vi "Fpga-Top-Level.vi"() -> ()   [LabVIEW 2016]
uses:
  <vilib>/Platform/TimedLoop/XDataNode/timing_clust.ctl
  <vilib>/Platform/TimedLoop/XDataNode/nitl_modes.ctl
  <vilib>/Platform/TimedLoop/XDataNode/wakeup.ctl
  <vilib>/rvi/Emulation/niFpgaSctlEmulationGetInTimedLoop.vi
  <vilib>/rvi/Emulation/niFpgaEmulationReportErrorSimple.vi
  <vilib>/rvi/Emulation/niFpgaGetClockAttributes.vi
  <vilib>/rvi/Emulation/niFpgaCriticalErrorInLSC.vi
  <vilib>/rvi/interface/RandomDataEmulation/niFpgaRandomDataHandleErrors.vi
  <vilib>/Platform/TimedLoop/XDataNode/XDataNode.xnode
  <vilib>/rvi/DataTransferAndStorage/Container/XNode/niFpgaContainer.xnode
  <vilib>/rvi/interface/RandomDataEmulation/nirviRandomDataFpgaReadWriteTemplate.vi
  <vilib>/Platform/TimedLoop/XDataNode/XDNodeRunTimeDep.lvlib
panel:
  out "Seconds":u32 format="%.0x"
  out "MsgType":u8
  out "MsgLen (16)":u16
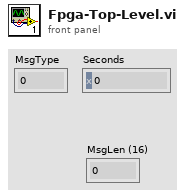
[diagram p1: front panel]
types:
  T1 = typedef "XDNodeRunTimeDep.lvlib/timing_clust.ctl" = cluster{"Expected End [f-1]":u64, "Actual End [f-1]":u64, "Finished Late? [f-1]":bool, "Expected End [i-1]":u64, "Actual End [i-1]":u64, "Finished Late? [i-1]":bool, "Expected Start [i]":u64, "Actual Start [i]":u64, "Expected Start [f]":u64, "Actual Start [f]":u64, "Source Name":string, "Structure Name":string, "Period":i64, "Deadline":i64, "Offset":i64, "Start":i64, "Priority":i32, "Timeout":i32, "Mode":T2, "Wakeup Reason":T3, "Error":errorcluster, "Source Type":string, "Secondary Source Type":string, "Global End Time":u64, "Global Start Time":u64, "Frame Duration":u64, "Iteration Duration":u64, "Assigned CPU":i32, "I/O Scan Engine Mode":u32}
  T2 = typedef "XDNodeRunTimeDep.lvlib/nitl_modes.ctl" = enum32{"No Change", "Process missed periods, maintain original phase", "Discard missed periods, maintain original phase", "Process missed periods, ignore original phase", "Discard missed periods, ignore original phase"}
  T3 = typedef "XDNodeRunTimeDep.lvlib/wakeup.ctl" = enum32{"Normal", "Aborted", "Asynchronous wakeup", "Timing source error", "Timed loop error", "Timeout"}
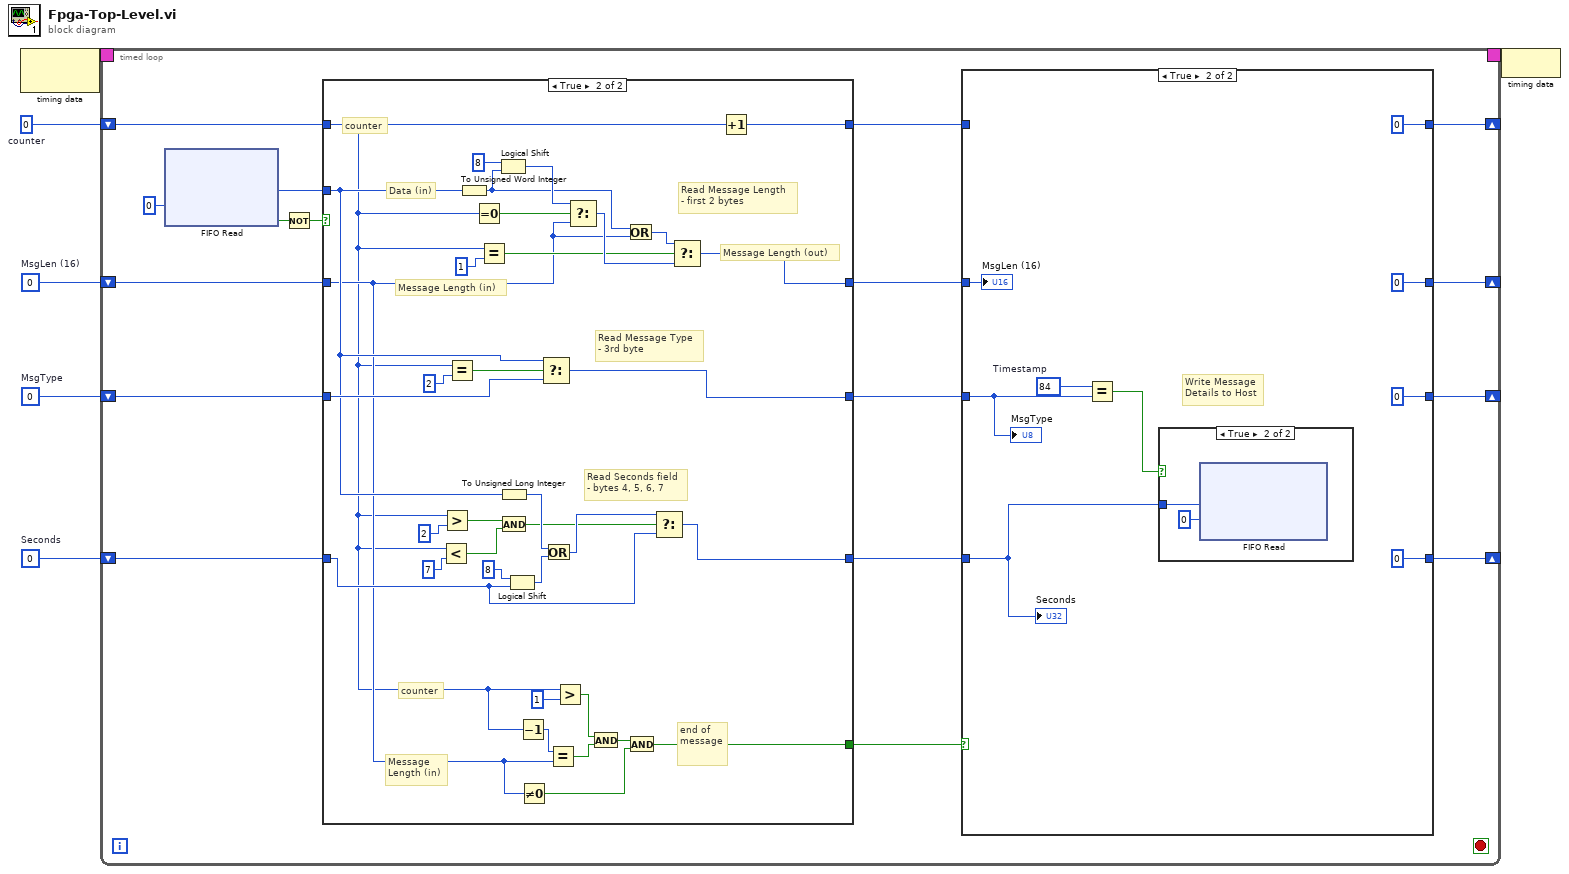
[diagram p0: block diagram]
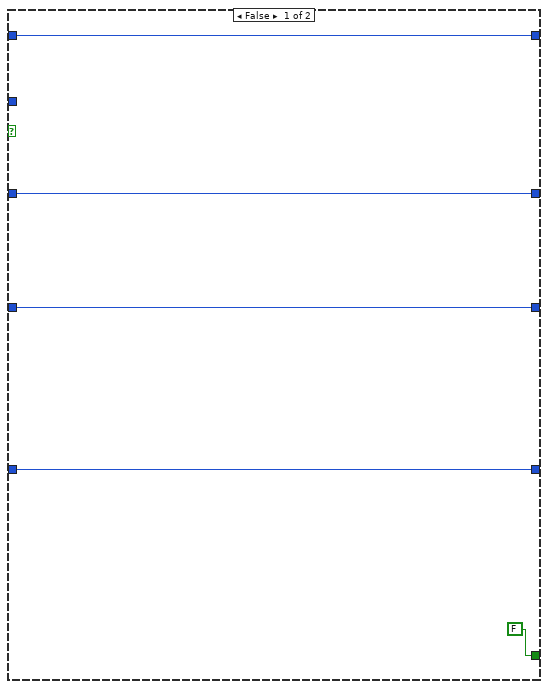
[diagram p4: hidden frame]
diagram:
  w1 = u32 0  # Seconds
  w2 = u8 0  # MsgType
  w3 = u16 0  # counter
  w4 = u16 0  # MsgLen (16)
  n1 = node-c288() -> (w6:T1)  [unwired: 1 in]
  n2 = timed-loop {
    timing: w6 -> [_]
    timing-out: [_] -> w5
    shift-right: [w12] -> _
    shift-left: w4 -> [w19]
    shift-right: [w13] -> _
    shift-left: w3 -> [w18]
    shift-right: [w10] -> _
    shift-left: w2 -> [w17]
    shift-right: [w8] -> _
    shift-left: w1 -> [w16]
    stop <- _ stop-if-true
    n3 = xnode ("FIFO Read")("Timeout"=0) -> ("Element"=w20:u8, "Timed Out?"=w22:bool)  [unwired: 1 in, 1 out]
    n4 = Not(x=w22) -> (.not. x?=w21:bool)
    n5 = case shown="True" w21 {
      tunnel: w20 -> [_ w49]
      tunnel: [w43 w73] -> w11
      tunnel: w19 -> [w43 w45]
      tunnel: w18 -> [w42 w44]
      tunnel: [w42 w77] -> w14
      tunnel: w17 -> [w41 w63]
      tunnel: [w41 w61] -> w9
      tunnel: w16 -> [w40 w50]
      tunnel: [w40 w59] -> w7
      tunnel: [FALSE w46] -> w15
      frame False {
      }
      frame True {
        # "Message\nLength (in)"
        # "counter"
        # "counter"
        # "Data (in)"
        # "Message Length (in)"
        # "Message Length (out)"
        # "Read Seconds field\n- bytes 4, 5, 6, 7"
        # "Read Message Type\n- 3rd byte"
        # "Read Message Length\n- first 2 bytes"
        # "end of\nmessage"
        n6 = Less?(x=w44, y=u16 7) -> (x < y?=w51:bool)
        n7 = Greater?(x=w44, y=u16 2) -> (0:w53:bool)
        n8 = Equal?(x=w44, y=u16 2) -> (x = y?=w62:bool)
        n9 = To Unsigned Word Integer(number=w49) -> (unsigned 16bit integer=w69:u16)
        n10 = Equal To 0?(x=w44) -> (x = 0?=w76:bool)
        n11 = Equal?(x=w44, y=u16 1) -> (x = y?=w74:bool)
        n12 = Logical Shift(y=i16 8, x=w69) -> (x << y=w70:u16)
        n13 = To Unsigned Long Integer(number=w49) -> (unsigned 32bit integer=w55:u32)
        n14 = And(x=w53, y=w51) -> (x .and. y?=w54:bool)
        n15 = Logical Shift(y=i16 8, x=w50) -> (x << y=w58:u32)
        n16 = Decrement(x=w44) -> (x-1=w65:u16)
        n17 = Not Equal To 0?(x=w45) -> (x != 0?=w48:bool)
        n18 = Select(t=w49, s=w62, f=w63) -> (s? t:f=w61:u8)
        n19 = Or(x=w55, y=w58) -> (x .or. y?=w57:u32)
        n20 = Equal?(x=w65, y=w45) -> (x = y?=w66:bool)
        n21 = Greater?(x=w44, y=u16 1) -> (0:w67:bool)
        n22 = Select(t=w70, s=w76, f=w45) -> (s? t:f=w75:u16)
        n23 = And(x=w67, y=w66) -> (x .and. y?=w47:bool)
        n24 = Or(x=w69, y=w45) -> (x .or. y?=w72:u16)
        n25 = And(x=w47, y=w48) -> (x .and. y?=w46:bool)
        n26 = Select(t=w57, s=w54, f=w50) -> (s? t:f=w59:u32)
        n27 = Select(t=w72, s=w74, f=w75) -> (s? t:f=w73:u16)
        n28 = Increment(x=w44) -> (x+1=w77:u16)
      }
    }
    n29 = case shown="True" w15 {
      tunnel: w14 -> [w24 _]
      tunnel: [w24 u16 0 ("counter")] -> w13
      tunnel: [w25 u16 0 ("MsgLen (16)")] -> w12
      tunnel: w11 -> [w25 w36]
      tunnel: [w26 u8 0 ("MsgType")] -> w10
      tunnel: w9 -> [w26 w30]
      tunnel: [w27 u32 0 ("Seconds")] -> w8
      tunnel: w7 -> [w27 w35]
      frame False {
      }
      frame True {
        w29 = u8 84  # Timestamp
        # "Write Message\nDetails to Host"
        n30 = Equal?(x=w29, y=w30) -> (x = y?=w28:bool)
        n31 = case shown="True" w28 {
          tunnel: w35 -> [_ w37]
          frame False {
          }
          frame True {
            n32 = xnode ("FIFO Read")("Element"=w37, "Timeout"=0) -> ()  [unwired: 1 in, 2 out]
          }
        }
        "MsgLen (16)" <- w36
        "MsgType" <- w30
        "Seconds" <- w35
      }
    }
  }
  n33 = node-c288(w5) -> ()
